vi "Update UI Status.vi"(7 "Previous Complete":bool, 8 "error in":errorcluster, 10 "Status to Display":string, 11 "String in":refnum<vi>) -> (0 "error out":errorcluster)   [LabVIEW 2021, in "Plugin Generator.lvlib"]
uses:
  CIF_Plugin_Generator.lvclass/CIF_Plugin_Generator.ctl
  Plugin Generator.lvlib
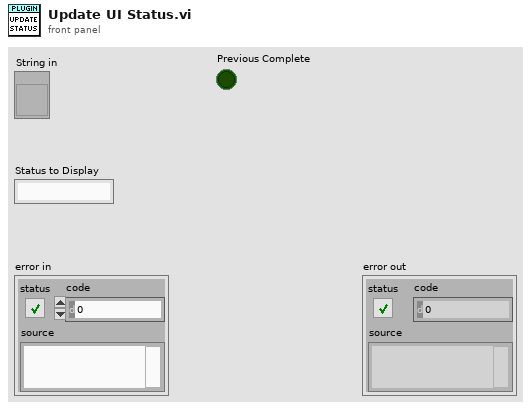
[diagram p1: front panel]
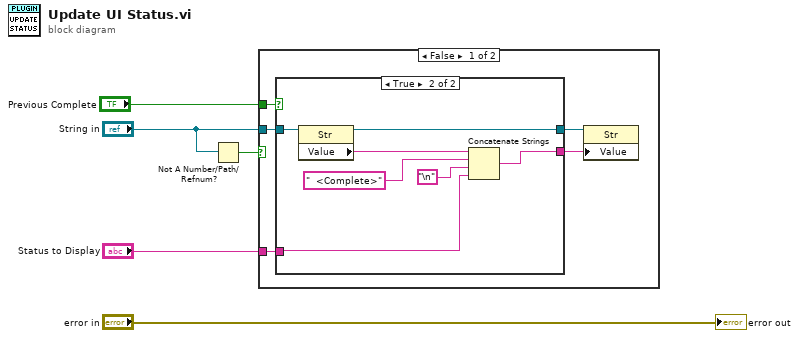
[diagram p0: block diagram]
diagram:
  n1 = Not A Number/Path/Refnum?(number/path/refnum="String in") -> (NaN/Path/Refnum?=w3:bool)
  n2 = case shown="False" w3 {
    tunnel: "String in" -> [w10 _]
    tunnel: "Status to Display" -> [w8 _]
    tunnel: "Previous Complete" -> [w7 _]
    frame False {
      n3 = case shown="True" w7 {
        tunnel: w10 -> [w11 w19]
        tunnel: [w11 w18] -> w9
        tunnel: w8 -> [w12 w14]
        tunnel: [w12 w13] -> w6
        frame False {
        }
        frame True {
          n4 = property class="Str"(reference=w19) -> (reference out=w18:refnum<vi>, "Value"=w17:string)  [unwired: 1 in, 1 out]
          n5 = Concatenate Strings(w17, "  <Complete>", "\n", w14) -> (w13:string)
        }
      }
      n6 = property class="Str"(reference=w9, "Value"=w6) -> ()  [unwired: 1 in, 2 out]
    }
    frame True {
    }
  }
  "error out" <- "error in"
